vi "findNode.vi"(0 "reference":refnum<class "Graph.lvclass">, 1 "point2D":T1 {"y" format="%.2f"; "x" format="%.2f"}, 2 "IgnoreTheseNodes":refnum<class "AbstractNode.lvclass">[](array[class]), 5 "error in (no error)":errorcluster) -> (14 "reference out":refnum<class "Graph.lvclass">, 15 "node":refnum<class "AbstractNode.lvclass">, 16 "found":bool, 19 "error out":errorcluster)   [LabVIEW 2014, in "Graph.lvclass"]
doc: "Finds a node containing the given point.\n @param p a point\n @return a node containing p or null if no nodes contain p\n */\n public Node findNode(Point2D p)"
uses:
  <resource>/Framework/Providers/Open_GDS/UML/Graph_class/Graph.lvclass
  <resource>/Framework/Providers/Open_GDS/UML/General/Point/Point Point2D.ctl
  <resource>/Framework/Providers/Open_GDS/UML/AbstractNode_class/AbstractNode.lvclass
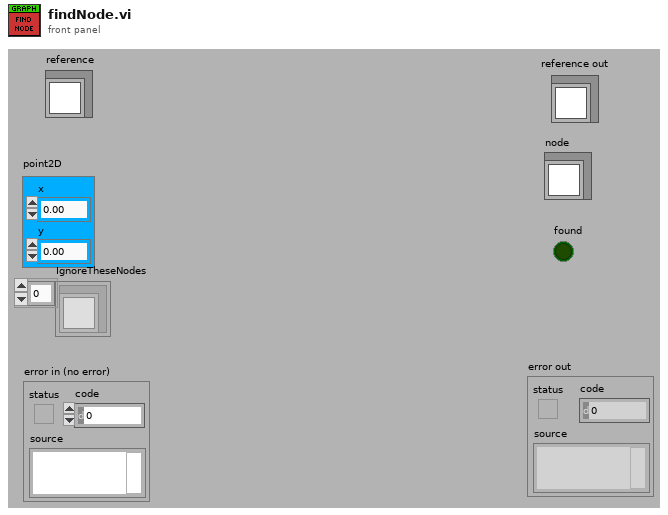
[diagram p1: front panel]
types:
  T1 = typedef "Point Point2D.ctl" = cluster{"x":dbl, "y":dbl}
  T2 = typedef "Graph.lvclass/ObjectAttributes.ctl" = cluster{"nodes":refnum<class "AbstractNode.lvclass">[], "edges":refnum<class "AbstractEdge.lvclass">[], "nodesToBeRemoved":refnum<class "AbstractNode.lvclass">[], "edgesToBeRemoved":refnum<class "AbstractEdge.lvclass">[], "needsLayout":bool, "LayoutNodes":refnum<class "AbstractNode.lvclass">[]}
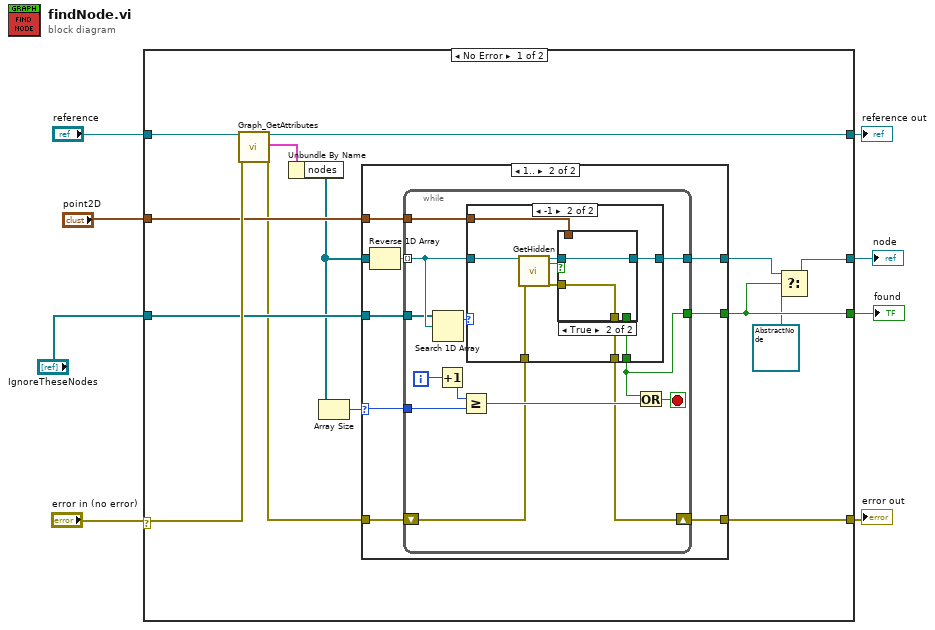
[diagram p0: block diagram]
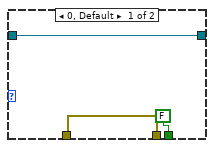
[diagram p3: hidden frame]
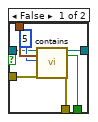
[diagram p4: hidden frame]
diagram:
  n1 = case shown="No Error" "error in (no error)" {
    selector: "error in (no error)" -> [w19 w67]
    tunnel: "reference" -> [w22 w68]
    tunnel: [w21 w67] -> w7
    tunnel: [w20 w68] -> w6
    tunnel: "point2D" -> [w18 _]
    tunnel: [w17 _] -> w3
    tunnel: [w16 _] -> w2
    tunnel: "IgnoreTheseNodes" -> [w15 _]
    frame No Error {
      n2 = call <resource>:"Graph_GetAttributes.vi"("reference in"=w22, "error in (no error)"=w19) -> ("reference out"=w20:refnum<class "Graph.lvclass">, "Attributes"=w14:T2, "error out"=w12:errorcluster)  [unwired: 15 out]
      n3 = Unbundle By Name(w14) -> ("nodes"=w13:refnum<class "AbstractNode.lvclass">[])
      n4 = Array Size(array=w13) -> (size(s)=w11:i32)
      n5 = case shown="1.." w11 {
        selector: w11 -> [_ w25]
        tunnel: w13 -> [_ w32]
        tunnel: w12 -> [w23 w31]
        tunnel: [w23 w30] -> w21
        tunnel: [_ w29] -> w10
        tunnel: w18 -> [_ w28]
        tunnel: [_ w27] -> w16
        tunnel: w15 -> [_ w24]
        frame 0, Default {
        }
        frame 1.. {
          n6 = Reverse 1D Array(array=w32) -> (reversed array=w26:refnum<class "AbstractNode.lvclass">[])
          n7 = while {
            tunnel: w25 -> [w43]
            tunnel: w26 -> [w36] mode=indexing
            shift-right: [w39] -> w30
            shift-left: w31 -> [w40]
            tunnel: [w38] -> w29
            tunnel: w28 -> [w37]
            tunnel: [w33] -> w27
            tunnel: w24 -> [w35]
            i -> [w45]
            stop <- w41 stop-if-true
            n8 = Search 1D Array(1D array=w35, element=w36) -> (index of element=w34:i32)  [unwired: 1 out]
            n9 = Increment(x=w45) -> (x+1=w44:i32)
            n10 = Greater Or Equal?(x=w44, y=w43) -> (x >= y?=w42:bool)
            n11 = case shown="-1" w34 {
              tunnel: w40 -> [w47 w50]
              tunnel: [w47 w57] -> w39
              tunnel: [w48 w56] -> w38
              tunnel: w36 -> [w48 w53]
              tunnel: w37 -> [_ w55]
              tunnel: [FALSE ("contains") w54] -> w33
              frame 0, Default {
              }
              frame -1 {
                n12 = call-dynamic "GetHidden.vi"("reference in"=w53, "error in (no error)"=w50) -> ("reference out"=w52:refnum<class "AbstractNode.lvclass">, "Hidden"=w49:bool, "error out"=w51:errorcluster)  [unwired: 15 in]
                n13 = case shown="True" w49 {
                  tunnel: [w64 w66] -> w57
                  tunnel: [w63 w65] -> w56
                  tunnel: w55 -> [w62 _]
                  tunnel: [w61 _] -> w54
                  tunnel: w52 -> [w59 w65]
                  tunnel: w51 -> [w58 w66]
                  frame False {
                    n14 = call-dynamic "contains.vi"("reference"=w59, "point2D"=w62, "AdditionalMargin"=5, "error in (no error)"=w58) -> ("reference out"=w63:refnum<class "AbstractNode.lvclass">, "contains"=w61:bool, "error out"=w64:errorcluster)  [unwired: 13 in]
                  }
                  frame True {
                  }
                }
              }
            }
            n15 = Or(x=w33, y=w42) -> (x .or. y?=w41:bool)
          }
        }
      }
      n16 = Select(t=w10, s=w16, f=refnum<class "AbstractNode.lvclass"> refnum) -> (s? t:f=w17:refnum<class "AbstractNode.lvclass">)
    }
    frame Error {
    }
  }
  "reference out" <- w6
  "error out" <- w7
  "found" <- w2
  "node" <- w3
